vi "counter 2 with semaphore.vi"() -> ()   [LabVIEW 2009]
panel:
  out "Compte total":i32
  out "Compte 2":i32
  out "total cumulatif":i32
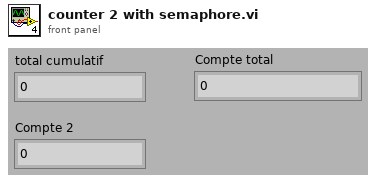
[diagram p1: front panel]
types:
  T1 = typedef "Semaphore RefNum" = refnum<k1>
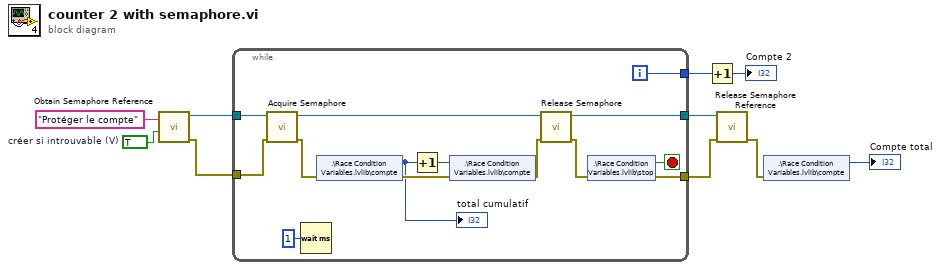
[diagram p0: block diagram]
diagram:
  w1 = TRUE  # créer si introuvable (V)
  n1 = call <vilib>:"Obtain Semaphore Reference.vi"("create if not found (T)"=w1, "name (unnamed)"="Protéger le compte") -> ("error out"=w6:errorcluster, "semaphore"=w7:T1)  [unwired: 3 in, 1 out]
  n2 = while "Boucle While" {
    tunnel: [w23] -> w10
    tunnel: w6 -> [w17]
    tunnel: [w22] -> w3
    tunnel: w7 -> [w18]
    tunnel: [w11] -> w2
    i -> [w23]
    stop <- w12 stop-if-true
    n3 = call <vilib>:"Acquire Semaphore.vi"("error in (no error)"=w17, "semaphore"=w18) -> ("error out"=w16:errorcluster, "semaphore out"=w13:T1)  [unwired: 3 in, 1 out]
    n4 = Wait (ms) ("Attendre (ms)")(milliseconds to wait=u32 1) -> ()  [unwired: 1 out]
    n5 = shared-variable ".\\Race Condition Variables.lvlib\\compte"(error in=w16) -> (w19:i32, error out=w24:errorcluster)
    "total cumulatif" <- w19
    n6 = Increment ("Incrémenter")(x=w19) -> (x+1=w20:i32)
    n7 = shared-variable ".\\Race Condition Variables.lvlib\\compte"(w20, error in=w24) -> (error out=w15:errorcluster)
    n8 = call <vilib>:"Release Semaphore.vi"("error in (no error)"=w15, "semaphore"=w13) -> ("error out"=w14:errorcluster, "semaphore out"=w11:T1)  [unwired: 4 in]
    n9 = shared-variable ".\\Race Condition Variables.lvlib\\stop"(error in=w14) -> (w12:bool, error out=w22:errorcluster)
  }
  n10 = Increment ("Incrémenter")(x=w10) -> (x+1=→"Compte 2":i32)
  n11 = call <vilib>:"Release Semaphore Reference.vi"("error in (no error)"=w3, "semaphore"=w2) -> ("error out"=w5:errorcluster)  [unwired: 8 in, 1 out]
  n12 = shared-variable ".\\Race Condition Variables.lvlib\\compte"(error in=w5) -> (→"Compte total":i32)  [unwired: 1 out]
